vi "TTM Global.vi"() -> ()   [LabVIEW 2019]
panel:
  in  "LakeShore Address":string="12"
  in  "Edwards Address":string="08"
  in  "MKS270 Address":string="15"
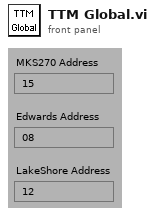
[diagram p1: front panel]
diagram:
